vi "Configure Pulse (Hold Paramter).vi"(8 "error in (no error)":errorcluster, 10 "Hold Parameter (Witdh)":enum16{"Width", "Duty Cycle"}(ring), 11 "VISA resource name":refnum<visa-resource-name>) -> (0 "error out":errorcluster, 3 "VISA resource name out":refnum<visa-resource-name>)   [LabVIEW 2017, in "Keithley 3390.lvlib"]
doc: "Sets the holf parameter of the pulse waveform."
uses:
  Keithley 3390.lvlib
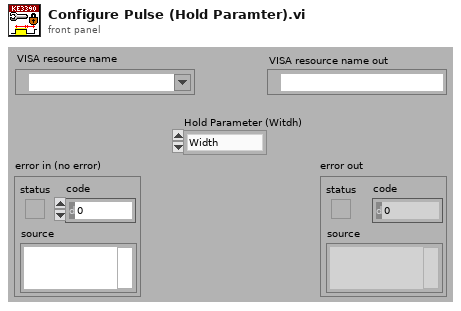
[diagram p1: front panel]
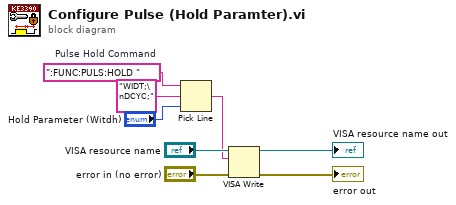
[diagram p0: block diagram]
diagram:
  w6 = ":FUNC:PULS:HOLD "  # Pulse Hold Command
  n1 = Pick Line(string ("")=w6, multi-line string="WIDT;\nDCYC;", line index="Hold Parameter (Witdh)") -> (output string=w3:string)
  n2 = VISA Write(VISA resource name="VISA resource name", write buffer=w3, error in (no error)="error in (no error)") -> (VISA resource name out=→"VISA resource name out":refnum<visa-resource-name>, error out=→"error out":errorcluster)  [unwired: 1 out]
